vi "Strip Offset mk2.vi"(8 "error in (no error)":errorcluster, 10 "Offset":u32, 11 "IFD in":refnum<class "IFD.lvclass">) -> (0 "error out":errorcluster, 3 "IFD out":refnum<class "IFD.lvclass">)   [LabVIEW 2016, in "IFD.lvclass"]
uses:
  IFD.lvclass
  IFD.lvclass/IFD.ctl
  Tag/IFD_Tag.lvclass/IFD_Tag.ctl
  Tag/IFD_Tag.lvclass
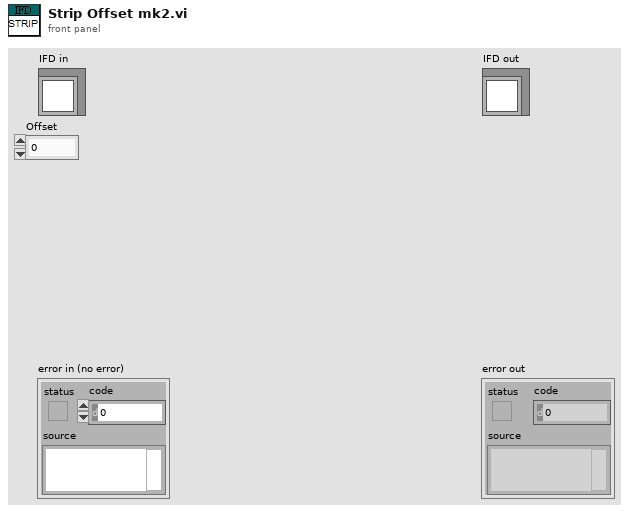
[diagram p1: front panel]
types:
  T1 = enum16{"big-endian, network order", "native, host order", "little-endian"}
  T2 = enum16{"Undefined(DO NOT USE)", "U8", "ASCII", "U16", "U32", "RATIONAL", "I8", "Undefined 8 bit", "I16", "I32", "SRATIONAL", "SGL", "DBL"}
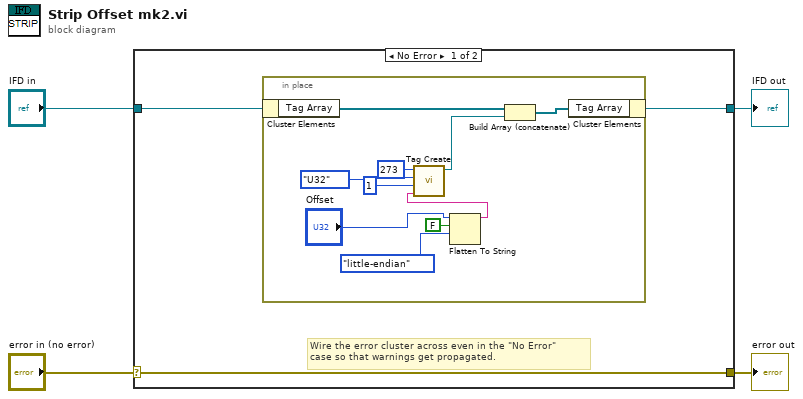
[diagram p0: block diagram]
diagram:
  n1 = case shown="No Error" "error in (no error)" {
    selector: "error in (no error)" -> [w7 w19]
    tunnel: [w7 w19] -> w3
    tunnel: [w5 w18] -> w1
    tunnel: "IFD in" -> [w6 w18]
    frame No Error {
      # "Wire the error cluster across even in the \"No Error\"\ncase so that warnings get propagated."
      n2 = in-place {
        n3 = in-place-cluster #1(w6) -> ("Tag Array"=w14:refnum<class "IFD_Tag.lvclass">[])
        n4 = Flatten To String(anything="Offset", prepend array or string size? (T)=FALSE, byte order (0:big-endian, network order)=T1."little-endian") -> (data string=w9:string)  [unwired: 1 in, 2 out]
        n5 = call "Tag Create.vi"("Data"=w9, "Data Count"=u32 1, "Data Type"=T2."U32", "Tag ID"=u16 273) -> ("IFD_Tag out"=w13:refnum<class "IFD_Tag.lvclass">)  [unwired: 7 in]
        n6 = Build Array (concatenate)(w14, w13) -> (w12:refnum<class "IFD_Tag.lvclass">[])
        n7 = in-place-cluster #1("Tag Array"=w12) -> (w5:refnum<class "IFD.lvclass">)
      }
    }
    frame Error {
    }
  }
  "error out" <- w3
  "IFD out" <- w1
